vi "MakeExample.vi"(8 "error in (no error)":errorcluster, 9 "TriggerRefractoryPeriod (Frames)":i32, 10 "StimulusObject Parameters":variant, 11 "JustTailRails in":refnum<class "JustTailRails.lvclass">) -> (0 "error out":errorcluster, 3 "JustTailRails out":refnum<class "JustTailRails.lvclass">)   [LabVIEW 2019, in "JustTailRails.lvclass"]
uses:
  JustTailRails.lvclass
  JustTailRailsInputCluster.ctl
  JustTailRails.lvclass/JustTailRails.ctl
  ParametersGlobal.vi
  StimulusObject.lvclass
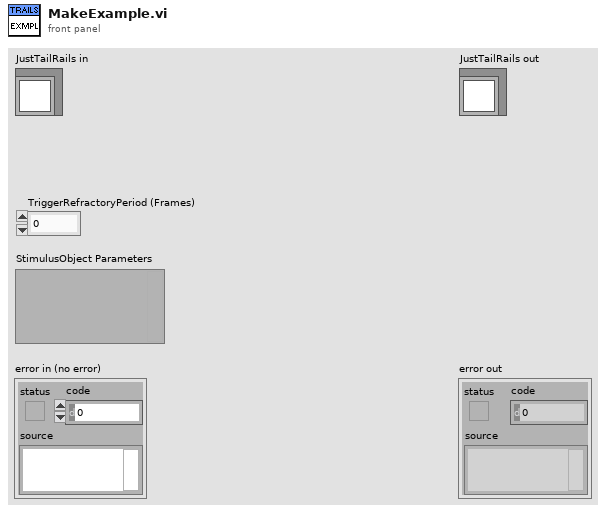
[diagram p1: front panel]
types:
  T1 = typedef "JustTailRails.lvclass/JustTailRailsInputCluster.ctl" = cluster{"Constant Intensity (uW/mm^2, negative is blue)":sgl, "dot radius (mm)":sgl, "Intensities (uW/mm^2, negative is blue)":sgl[], "Durations (s)":sgl[], "Inter trigger interval (s)":dbl}
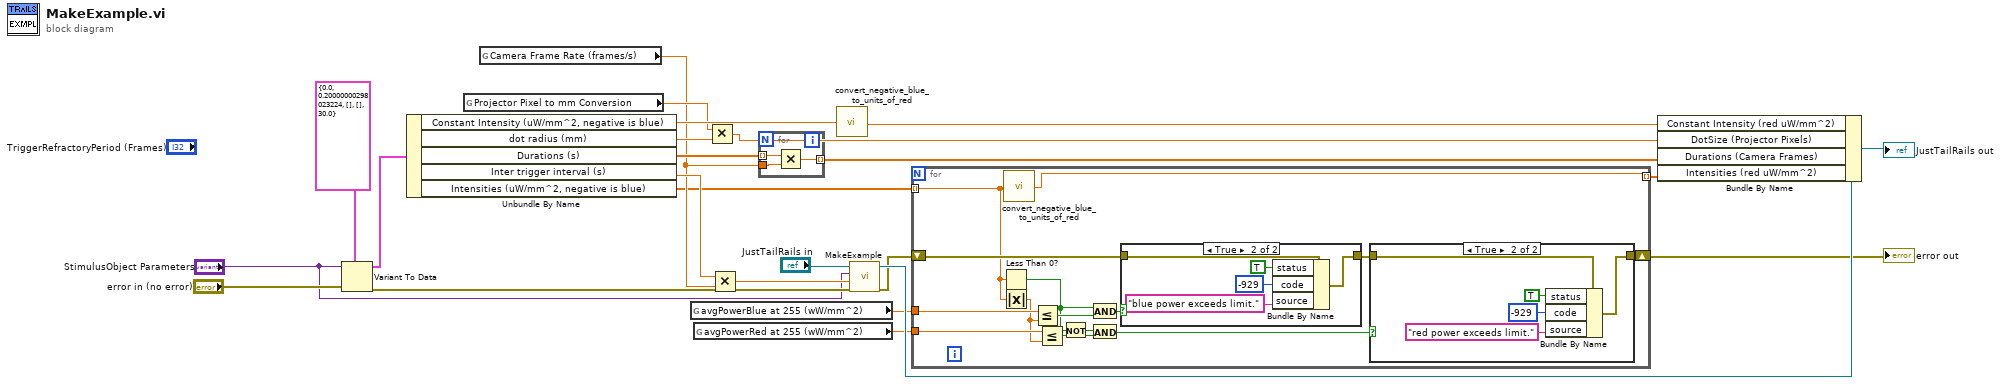
[diagram p0: block diagram]
diagram:
  n1 = Variant To Data(error in="error in (no error)", type=T1 {"Constant Intensity (uW/mm^2, negative is blue)"=0.0, "dot radius (mm)"=0.2, "Intensities (uW/mm^2, negative is blue)"=[], "Durations (s)"=[], "Inter trigger interval (s)"=30.0} ("JustHeadsRailsInputCluster"), Variant="StimulusObject Parameters") -> (data=w23:T1, error out=w24:errorcluster)
  n2 = Unbundle By Name(w23) -> ("Constant Intensity (uW/mm^2, negative is blue)"=w19:sgl, "dot radius (mm)"=w17:sgl, "Durations (s)"=w14:sgl[], "Inter trigger interval (s)"=w22:dbl, "Intensities (uW/mm^2, negative is blue)"=w11:sgl[])
  n3 = global read "ParametersGlobal.vi" "Projector Pixel to mm Conversion"() -> (w16:sgl)
  n4 = global read "ParametersGlobal.vi" "Camera Frame Rate (frames/s)"() -> (w13:sgl)
  n5 = global read "ParametersGlobal.vi" "avgPowerBlue at 255 (wW/mm^2)"() -> (w9:sgl)
  n6 = global read "ParametersGlobal.vi" "avgPowerRed at 255 (wW/mm^2)"() -> (w8:sgl)
  n7 = Multiply(x=w16, y=w17) -> (x*y=w15:sgl)
  n8 = Multiply(x=w22, y=w13) -> (x*y=w21:dbl)
  n9 = for {
    tunnel: w14 -> [w27] mode=indexing
    tunnel: w13 -> [w26]
    tunnel: [w25] -> w12 mode=indexing
    n10 = Multiply(x=w27, y=w26) -> (x*y=w25:sgl)
  }
  n11 = call "convert_negative_blue_to_units_of_red.vi"("Intensity in units of red (positive) and blue (negative)"=w19) -> ("Intensity in units of red (positive and negative)"=w18:sgl)
  n12 = call-parent "MakeExample.vi"("error in (no error)"=w24, "TriggerRefractoryPeriod (Frames)"=w21, "StimulusObject Parameters"="StimulusObject Parameters", "StimulusObject in"="JustTailRails in") -> ("error out"=w10:errorcluster, "StimulusObject out"=w20:refnum<class "JustTailRails.lvclass">)  [unwired: 6 in]
  n13 = for {
    tunnel: w11 -> [w35] mode=indexing
    shift-right: [w39] -> w2
    shift-left: w10 -> [w40]
    tunnel: w9 -> [w38]
    tunnel: w8 -> [w37]
    tunnel: [w36] -> w7 mode=indexing
    n14 = Less Than 0?(x=w35) -> (x < 0?=w28:bool)
    n15 = Absolute Value(x=w35) -> (abs(x)=w34:sgl)
    n16 = call "convert_negative_blue_to_units_of_red.vi"("Intensity in units of red (positive) and blue (negative)"=w35) -> ("Intensity in units of red (positive and negative)"=w36:sgl)
    n17 = Less Or Equal?(x=w38, y=w34) -> (x <= y?=w33:bool)
    n18 = Less Or Equal?(x=w37, y=w34) -> (x <= y?=w30:bool)
    n19 = Not(x=w28) -> (.not. x?=w29:bool)
    n20 = And(x=w28, y=w33) -> (x .and. y?=w32:bool)
    n21 = And(x=w29, y=w30) -> (x .and. y?=w31:bool)
    n22 = case shown="True" w32 {
      tunnel: w40 -> [w48 w53]
      tunnel: [w48 w52] -> w41
      frame False {
      }
      frame True {
        n23 = Bundle By Name(cluster=w53, "status"=TRUE, "code"=-929, "source"="blue power exceeds limit.") -> (w52:errorcluster)
      }
    }
    n24 = case shown="True" w31 {
      tunnel: w41 -> [w42 w47]
      tunnel: [w42 w46] -> w39
      frame False {
      }
      frame True {
        n25 = Bundle By Name(cluster=w47, "status"=TRUE, "code"=-929, "source"="red power exceeds limit.") -> (w46:errorcluster)
      }
    }
  }
  "error out" <- w2
  n26 = Bundle By Name(cluster=w20, "Constant Intensity (red uW/mm^2)"=w18, "DotSize (Projector Pixels)"=w15, "Durations (Camera Frames)"=w12, "Intensities (red uW/mm^2)"=w7) -> (→"JustTailRails out":refnum<class "JustTailRails.lvclass">)
